vi "HFRR ADV v016 new software.vi"() -> ()   [LabVIEW 2025] (continued)
              tunnel: w2019 -> [w2034]
              i -> [w2030]
              stop <- w2029 continue-if-true
              (unwired) TRUE ("line mode (F)")
              n2041 = Read from Text File "Read File"(file (use dialog)=w2034) -> (text=w2031:string)  [unwired: 3 in, 3 out]
              n2042 = local write "Numeric 8"(w2030) -> ()
              n2043 = String Length(string=w2031) -> (length=w2033:i32)
              n2044 = Greater?(x=w2033, y=1) -> (0:w2029:bool)
            }
          }
          frame #1 {
            w2204 = FALSE ("ACTUAL   MERGE")
            # "Sample Temp"
            # "ECR"
            # "COF"
            # "Time\nCOF\nFF\nTemp"
            n2045 = case shown="True" w2077 {
              tunnel: [w2224 w2225] -> w2078
              frame False {
                n2046 = local read "string1"() -> (w2224:string)
              }
              frame True {
                n2047 = local read "String Indicator 4"() -> (w2225:string)
              }
            }
            n2048 = local read "string1 3"() -> (w2122:string)
            n2049 = String To Path(string=w2078) -> (path=w2209:path)
            n2050 = String To Path(string=w2122) -> (path=w2220:path)
            n2051 = local read "Numeric 12"() -> (w2206:i32)
            n2052 = local read "Numeric 8"() -> (w2208:i32)
            n2053 = local read "string1 2"() -> (w2123:string)
            n2054 = local read "string1 4"() -> (w2121:string)
            n2055 = Open/Create/Replace File "Open File"(file path (use dialog)=w2209) -> (refnum out=w2223:refnum<file>, error out=w2222:errorcluster)  [unwired: 5 in, 1 out]
            n2056 = Open/Create/Replace File "Open File"(file path (use dialog)=w2220) -> (refnum out=w2216:refnum<file>, error out=w2217:errorcluster)  [unwired: 5 in, 1 out]
            n2057 = for {
              N: w2208 -> [_]
              tunnel: w2223 -> [w2371]
              tunnel: w2222 -> [w2370]
              tunnel: [w2360] -> w2135 mode=indexing
              tunnel: [w2358] -> w2192 mode=indexing
              tunnel: [w2359] -> w2187 mode=indexing
              tunnel: w2204 -> [_]
              tunnel: [w2352] -> w2189 mode=indexing
              tunnel: [w2348] -> w2158 mode=indexing
              tunnel: [w2344] -> w2133 mode=indexing
              tunnel: [w2340] -> w2114 mode=indexing
              tunnel: [w2335] -> w2074 mode=indexing
              (unwired) TRUE ("line mode (F)")
              # "freq"
              # "Stroke"
              # "Time"
              # "CoF"
              # "Humidity"
              # "Temp"
              # "Air Temp"
              # "ECR"
              n2058 = Read from Text File "Read File"(file (use dialog)=w2371, error in=w2370) -> (text=w2336:string)  [unwired: 2 in, 3 out]
              n2059 = local write "String 6"(w2336) -> ()
              n2060 = String Subset(string=w2336, offset (0)=0, length (rest)=14 ("length (rest)")) -> (substring=w2364:string)
              n2061 = String Subset(string=w2336, offset (0)=35, length (rest)=9 ("length (rest)")) -> (substring=w2361:string)
              n2062 = String Subset(string=w2336, offset (0)=15, length (rest)=9 ("length (rest)")) -> (substring=w2367:string)
              n2063 = Fract/Exp String To Number(string=w2364) -> (number=w2360:dbl)  [unwired: 3 in, 1 out]
              n2064 = Fract/Exp String To Number(string=w2361) -> (number=w2359:dbl)  [unwired: 3 in, 1 out]
              n2065 = Fract/Exp String To Number(string=w2367) -> (number=w2358:dbl)  [unwired: 3 in, 1 out]
              n2066 = String Subset(string=w2336, offset (0)=85, length (rest)=9 ("length (rest)")) -> (substring=w2337:string)
              n2067 = String Subset(string=w2336, offset (0)=25, length (rest)=9 ("length (rest)")) -> (substring=w2343:string)
              n2068 = String Subset(string=w2336, offset (0)=55, length (rest)=9 ("length (rest)")) -> (substring=w2345:string)
              n2069 = String Subset(string=w2336, offset (0)=45, length (rest)=9 ("length (rest)")) -> (substring=w2351:string)
              n2070 = String Subset(string=w2336, offset (0)=65, length (rest)=9 ("length (rest)")) -> (substring=w2357:string)
              n2071 = Fract/Exp String To Number(string=w2343) -> (number=w2340:dbl)  [unwired: 3 in, 1 out]
              n2072 = Fract/Exp String To Number(string=w2337) -> (number=w2335:dbl)  [unwired: 3 in, 1 out]
              n2073 = Fract/Exp String To Number(string=w2345) -> (number=w2344:dbl)  [unwired: 3 in, 1 out]
              n2074 = Fract/Exp String To Number(string=w2351) -> (number=w2348:dbl)  [unwired: 3 in, 1 out]
              n2075 = Fract/Exp String To Number(string=w2357) -> (number=w2354:dbl)  [unwired: 3 in, 1 out]
              n2076 = Add(x=w2354, y=0.0) -> (x+y=w2352:dbl)
            }
            n2077 = for {
              N: w2206 -> [_]
              tunnel: w2217 -> [w2297]
              tunnel: w2216 -> [w2296]
              tunnel: [w2286] -> w2175 mode=indexing
              tunnel: [w2284] -> w2173 mode=indexing
              tunnel: [w2285] -> w2169 mode=indexing
              tunnel: w2204 -> [_]
              tunnel: [w2278] -> w2171 mode=indexing
              tunnel: [w2274] -> w2153 mode=indexing
              tunnel: [w2270] -> w2129 mode=indexing
              tunnel: [w2267] -> w2110 mode=indexing
              tunnel: [w2263] -> w2069 mode=indexing
              (unwired) 9 ("length (rest)")
              (unwired) 9 ("length (rest)")
              (unwired) TRUE ("line mode (F)")
              n2078 = Read from Text File "Read File"(file (use dialog)=w2296, error in=w2297) -> (text=w2264:string)  [unwired: 2 in, 3 out]
              n2079 = local write "String 8"(w2264) -> ()
              n2080 = String Subset(string=w2264, offset (0)=85) -> (substring=w2266:string)  [unwired: 1 in]
              n2081 = String Subset(string=w2264, offset (0)=35, length (rest)=9 ("length (rest)")) -> (substring=w2287:string)
              n2082 = String Subset(string=w2264, offset (0)=55, length (rest)=9 ("length (rest)")) -> (substring=w2272:string)
              n2083 = String Subset(string=w2264, offset (0)=25) -> (substring=w2268:string)  [unwired: 1 in]
              n2084 = String Subset(string=w2264, offset (0)=15, length (rest)=9 ("length (rest)")) -> (substring=w2293:string)
              n2085 = String Subset(string=w2264, offset (0)=0, length (rest)=14 ("length (rest)")) -> (substring=w2290:string)
              n2086 = String Subset(string=w2264, offset (0)=45, length (rest)=9 ("length (rest)")) -> (substring=w2277:string)
              n2087 = String Subset(string=w2264, offset (0)=65, length (rest)=9 ("length (rest)")) -> (substring=w2283:string)
              n2088 = Fract/Exp String To Number(string=w2266) -> (number=w2263:dbl)  [unwired: 3 in, 1 out]
              n2089 = Fract/Exp String To Number(string=w2287) -> (number=w2285:dbl)  [unwired: 3 in, 1 out]
              n2090 = Fract/Exp String To Number(string=w2272) -> (number=w2270:dbl)  [unwired: 3 in, 1 out]
              n2091 = Fract/Exp String To Number(string=w2268) -> (number=w2267:dbl)  [unwired: 3 in, 1 out]
              n2092 = Fract/Exp String To Number(string=w2293) -> (number=w2284:dbl)  [unwired: 3 in, 1 out]
              n2093 = Fract/Exp String To Number(string=w2290) -> (number=w2286:dbl)  [unwired: 3 in, 1 out]
              n2094 = Fract/Exp String To Number(string=w2277) -> (number=w2274:dbl)  [unwired: 3 in, 1 out]
              n2095 = Fract/Exp String To Number(string=w2283) -> (number=w2280:dbl)  [unwired: 3 in, 1 out]
              n2096 = Add(x=w2280, y=0.0) -> (x+y=w2278:dbl)
            }
            n2097 = String To Path(string=w2123) -> (path=w2221:path)
            n2098 = String To Path(string=w2121) -> (path=w2215:path)
            n2099 = local read "Numeric 11"() -> (w2205:i32)
            n2100 = local read "Numeric 13"() -> (w2207:i32)
            n2101 = Open/Create/Replace File "Open File"(file path (use dialog)=w2221) -> (refnum out=w2219:refnum<file>, error out=w2218:errorcluster)  [unwired: 5 in, 1 out]
            n2102 = Open/Create/Replace File "Open File"(file path (use dialog)=w2215) -> (refnum out=w2214:refnum<file>, error out=w2213:errorcluster)  [unwired: 5 in, 1 out]
            n2103 = for {
              N: w2205 -> [_]
              tunnel: w2219 -> [w2334]
              tunnel: w2218 -> [w2333]
              tunnel: [w2323] -> w2185 mode=indexing
              tunnel: [w2321] -> w2183 mode=indexing
              tunnel: [w2322] -> w2178 mode=indexing
              tunnel: w2204 -> [_]
              tunnel: [w2315] -> w2180 mode=indexing
              tunnel: [w2311] -> w2156 mode=indexing
              tunnel: [w2307] -> w2131 mode=indexing
              tunnel: [w2303] -> w2112 mode=indexing
              tunnel: [w2298] -> w2070 mode=indexing
              (unwired) TRUE ("line mode (F)")
              n2104 = Read from Text File "Read File"(file (use dialog)=w2334, error in=w2333) -> (text=w2299:string)  [unwired: 2 in, 3 out]
              n2105 = local write "String 7"(w2299) -> ()
              n2106 = String Subset(string=w2299, offset (0)=85, length (rest)=9 ("length (rest)")) -> (substring=w2302:string)
              n2107 = String Subset(string=w2299, offset (0)=35, length (rest)=9 ("length (rest)")) -> (substring=w2324:string)
              n2108 = String Subset(string=w2299, offset (0)=55, length (rest)=9 ("length (rest)")) -> (substring=w2310:string)
              n2109 = String Subset(string=w2299, offset (0)=25, length (rest)=9 ("length (rest)")) -> (substring=w2304:string)
              n2110 = String Subset(string=w2299, offset (0)=45, length (rest)=9 ("length (rest)")) -> (substring=w2312:string)
              n2111 = String Subset(string=w2299, offset (0)=0, length (rest)=14 ("length (rest)")) -> (substring=w2327:string)
              n2112 = String Subset(string=w2299, offset (0)=15, length (rest)=9 ("length (rest)")) -> (substring=w2330:string)
              n2113 = String Subset(string=w2299, offset (0)=65, length (rest)=9 ("length (rest)")) -> (substring=w2316:string)
              n2114 = Fract/Exp String To Number(string=w2302) -> (number=w2298:dbl)  [unwired: 3 in, 1 out]
              n2115 = Fract/Exp String To Number(string=w2324) -> (number=w2322:dbl)  [unwired: 3 in, 1 out]
              n2116 = Fract/Exp String To Number(string=w2310) -> (number=w2307:dbl)  [unwired: 3 in, 1 out]
              n2117 = Fract/Exp String To Number(string=w2304) -> (number=w2303:dbl)  [unwired: 3 in, 1 out]
              n2118 = Fract/Exp String To Number(string=w2312) -> (number=w2311:dbl)  [unwired: 3 in, 1 out]
              n2119 = Fract/Exp String To Number(string=w2327) -> (number=w2323:dbl)  [unwired: 3 in, 1 out]
              n2120 = Fract/Exp String To Number(string=w2330) -> (number=w2321:dbl)  [unwired: 3 in, 1 out]
              n2121 = Fract/Exp String To Number(string=w2316) -> (number=w2319:dbl)  [unwired: 3 in, 1 out]
              n2122 = Add(x=w2319, y=0.0) -> (x+y=w2315:dbl)
            }
            n2123 = for {
              N: w2207 -> [_]
              tunnel: w2214 -> [w2262]
              tunnel: w2213 -> [w2261]
              tunnel: [w2251] -> w2167 mode=indexing
              tunnel: [w2250] -> w2160 mode=indexing
              tunnel: w2204 -> [_]
              tunnel: [w2239] -> w2165 mode=indexing
              tunnel: [w2244] -> w2162 mode=indexing
              tunnel: [w2240] -> w2152 mode=indexing
              tunnel: [w2235] -> w2127 mode=indexing
              tunnel: [w2231] -> w2108 mode=indexing
              tunnel: [w2226] -> w2068 mode=indexing
              (unwired) 1.0 ("x")
              (unwired) TRUE ("line mode (F)")
              n2124 = Read from Text File "Read File"(file (use dialog)=w2262, error in=w2261) -> (text=w2227:string)  [unwired: 2 in, 3 out]
              n2125 = local write "String 12"(w2227) -> ()
              n2126 = String Subset(string=w2227, offset (0)=85, length (rest)=9 ("length (rest)")) -> (substring=w2229:string)
              n2127 = String Subset(string=w2227, offset (0)=35, length (rest)=9 ("length (rest)")) -> (substring=w2252:string)
              n2128 = String Subset(string=w2227, offset (0)=55, length (rest)=9 ("length (rest)")) -> (substring=w2237:string)
              n2129 = String Subset(string=w2227, offset (0)=25, length (rest)=9 ("length (rest)")) -> (substring=w2233:string)
              n2130 = String Subset(string=w2227, offset (0)=45, length (rest)=9 ("length (rest)")) -> (substring=w2242:string)
              n2131 = String Subset(string=w2227, offset (0)=15, length (rest)=9 ("length (rest)")) -> (substring=w2258:string)
              n2132 = String Subset(string=w2227, offset (0)=0, length (rest)=14 ("length (rest)")) -> (substring=w2255:string)
              n2133 = String Subset(string=w2227, offset (0)=65, length (rest)=9 ("length (rest)")) -> (substring=w2245:string)
              n2134 = Fract/Exp String To Number(string=w2229) -> (number=w2226:dbl)  [unwired: 3 in, 1 out]
              n2135 = Fract/Exp String To Number(string=w2252) -> (number=w2250:dbl)  [unwired: 3 in, 1 out]
              n2136 = Fract/Exp String To Number(string=w2237) -> (number=w2235:dbl)  [unwired: 3 in, 1 out]
              n2137 = Fract/Exp String To Number(string=w2233) -> (number=w2231:dbl)  [unwired: 3 in, 1 out]
              n2138 = Fract/Exp String To Number(string=w2242) -> (number=w2240:dbl)  [unwired: 3 in, 1 out]
              n2139 = Fract/Exp String To Number(string=w2258) -> (number=w2239:dbl)  [unwired: 3 in, 1 out]
              n2140 = Fract/Exp String To Number(string=w2255) -> (number=w2251:dbl)  [unwired: 3 in, 1 out]
              n2141 = Fract/Exp String To Number(string=w2245) -> (number=w2248:dbl)  [unwired: 3 in, 1 out]
              n2142 = Add(x=w2248, y=0.0) -> (x+y=w2244:dbl)
            }
            n2143 = Delete From Array(array=w2110, index=0) -> (array with subset deleted=w2083:dbl[])  [unwired: 1 in, 1 out]
            n2144 = Delete From Array(array=w2173, index=0) -> (array with subset deleted=w2146:dbl[])  [unwired: 1 in, 1 out]
            n2145 = Delete From Array(array=w2153, index=0) -> (array with subset deleted=w2141:dbl[])  [unwired: 1 in, 1 out]
            n2146 = Delete From Array(array=w2171, index=0) -> (array with subset deleted=w2172:dbl[])  [unwired: 1 in, 1 out]
            n2147 = call-poly <vilib>:"Mean.vi"("X"=w2083) -> ("mean"=→"КОФ2 4":dbl)  [unwired: 1 out]
            n2148 = call-poly <vilib>:"Mean.vi"("X"=w2146) -> ("mean"=→"КОФ3":dbl)  [unwired: 1 out]
            n2149 = call-poly <vilib>:"Mean.vi"("X"=w2141) -> ("mean"=→"CP3":dbl)  [unwired: 1 out]
            n2150 = Delete From Array(array=w2135, index=0) -> (array with subset deleted=w2062:dbl[])  [unwired: 1 in, 1 out]
            n2151 = Delete From Array(array=w2074, index=0) -> (array with subset deleted=w2061:dbl[])  [unwired: 1 in, 1 out]
            n2152 = Delete From Array(array=w2114, index=0) -> (array with subset deleted=w2085:dbl[])  [unwired: 1 in, 1 out]
            n2153 = Delete From Array(array=w2192, index=0) -> (array with subset deleted=w2147:dbl[])  [unwired: 1 in, 1 out]
            n2154 = Delete From Array(array=w2158, index=0) -> (array with subset deleted=w2143:dbl[])  [unwired: 1 in, 1 out]
            "array w/ subset deleted" <- w2143
            n2155 = Delete From Array(array=w2189, index=0) -> (array with subset deleted=w2190:dbl[])  [unwired: 1 in, 1 out]
            n2156 = call-poly <vilib>:"Mean.vi"("X"=w2085) -> ("mean"=→"КОФ2 2":dbl)  [unwired: 1 out]
            n2157 = call-poly <vilib>:"Mean.vi"("X"=w2147) -> ("mean"=→"КОФ1":dbl)  [unwired: 1 out]
            n2158 = Bundle "Bundle"(w2062, w2061) -> (w2067:cluster{dbl[], dbl[]})  [unwired: 1 in]
            n2159 = Bundle "Bundle"(w2062, w2190) -> (w2054:cluster{dbl[], dbl[]})  [unwired: 1 in]
            n2160 = Delete From Array(array=w2069, index=0) -> (array with subset deleted=w2057:dbl[])  [unwired: 1 in, 1 out]
            n2161 = Delete From Array(array=w2070, index=0) -> (array with subset deleted=w2059:dbl[])  [unwired: 1 in, 1 out]
            n2162 = Delete From Array(array=w2180, index=0) -> (array with subset deleted=w2181:dbl[])  [unwired: 1 in, 1 out]
            n2163 = Delete From Array(array=w2068, index=0) -> (array with subset deleted=w2055:dbl[])  [unwired: 1 in, 1 out]
            n2164 = Delete From Array(array=w2162, index=0) -> (array with subset deleted=w2163:dbl[])  [unwired: 1 in, 1 out]
            n2165 = Delete From Array(array=w2187, index=0) -> (array with subset deleted=w2093:dbl[])  [unwired: 1 in, 1 out]
            n2166 = Delete From Array(array=w2133, index=0) -> (array with subset deleted=w2089:dbl[])  [unwired: 1 in, 1 out]
            n2167 = Delete From Array(array=w2169, index=0) -> (array with subset deleted=w2091:dbl[])  [unwired: 1 in, 1 out]
            n2168 = Delete From Array(array=w2129, index=0) -> (array with subset deleted=w2087:dbl[])  [unwired: 1 in, 1 out]
            n2169 = Delete From Array(array=w2178, index=0) -> (array with subset deleted=w2092:dbl[])  [unwired: 1 in, 1 out]
            n2170 = Delete From Array(array=w2131, index=0) -> (array with subset deleted=w2088:dbl[])  [unwired: 1 in, 1 out]
            n2171 = Delete From Array(array=w2112, index=0) -> (array with subset deleted=w2084:dbl[])  [unwired: 1 in, 1 out]
            n2172 = Delete From Array(array=w2156, index=0) -> (array with subset deleted=w2142:dbl[])  [unwired: 1 in, 1 out]
            n2173 = Delete From Array(array=w2183, index=0) -> (array with subset deleted=w2144:dbl[])  [unwired: 1 in, 1 out]
            n2174 = Delete From Array(array=w2160, index=0) -> (array with subset deleted=w2090:dbl[])  [unwired: 1 in, 1 out]
            n2175 = Delete From Array(array=w2127, index=0) -> (array with subset deleted=w2086:dbl[])  [unwired: 1 in, 1 out]
            n2176 = Delete From Array(array=w2108, index=0) -> (array with subset deleted=w2082:dbl[])  [unwired: 1 in, 1 out]
            n2177 = Delete From Array(array=w2152, index=0) -> (array with subset deleted=w2140:dbl[])  [unwired: 1 in, 1 out]
            n2178 = Delete From Array(array=w2165, index=0) -> (array with subset deleted=w2145:dbl[])  [unwired: 1 in, 1 out]
            n2179 = Delete From Array(array=w2175, index=0) -> (array with subset deleted=w2058:dbl[])  [unwired: 1 in, 1 out]
            n2180 = Delete From Array(array=w2185, index=0) -> (array with subset deleted=w2060:dbl[])  [unwired: 1 in, 1 out]
            n2181 = Delete From Array(array=w2167, index=0) -> (array with subset deleted=w2056:dbl[])  [unwired: 1 in, 1 out]
            n2182 = Bundle "Bundle"(w2062, w2093) -> (w2080:cluster{dbl[], dbl[]})  [unwired: 1 in]
            n2183 = Bundle "Bundle"(w2062, w2147) -> (w2081:cluster{dbl[], dbl[]})  [unwired: 1 in]
            n2184 = Bundle "Bundle"(w2093, w2089) -> (w2095:cluster{dbl[], dbl[]})  [unwired: 1 in]
            n2185 = Bundle "Bundle"(w2058, w2057) -> (w2065:cluster{dbl[], dbl[]})  [unwired: 1 in]
            n2186 = Bundle "Bundle"(w2091, w2087) -> (w2097:cluster{dbl[], dbl[]})  [unwired: 1 in]
            n2187 = Bundle "Bundle"(w2058, w2091) -> (w2201:cluster{dbl[], dbl[]})  [unwired: 1 in]
            n2188 = Bundle "Bundle"(w2058, w2087) -> (w2125:cluster{dbl[], dbl[]})  [unwired: 1 in]
            n2189 = Bundle "Bundle"(w2058, w2146) -> (w2211:cluster{dbl[], dbl[]})  [unwired: 1 in]
            n2190 = Bundle "Bundle"(w2058, w2141) -> (w2149:cluster{dbl[], dbl[]})  [unwired: 1 in]
            n2191 = Bundle "Bundle"(w2058, w2172) -> (w2196:cluster{dbl[], dbl[]})  [unwired: 1 in]
            n2192 = Bundle "Bundle"(w2092, w2088) -> (w2096:cluster{dbl[], dbl[]})  [unwired: 1 in]
            n2193 = Bundle "Bundle"(w2060, w2059) -> (w2066:cluster{dbl[], dbl[]})  [unwired: 1 in]
            n2194 = Bundle "Bundle"(w2060, w2092) -> (w2203:cluster{dbl[], dbl[]})  [unwired: 1 in]
            n2195 = Bundle "Bundle"(w2060, w2088) -> (w2126:cluster{dbl[], dbl[]})  [unwired: 1 in]
            n2196 = Bundle "Bundle"(w2060, w2142) -> (w2150:cluster{dbl[], dbl[]})  [unwired: 1 in]
            n2197 = Bundle "Bundle"(w2060, w2144) -> (w2212:cluster{dbl[], dbl[]})  [unwired: 1 in]
            n2198 = Bundle "Bundle"(w2060, w2181) -> (w2194:cluster{dbl[], dbl[]})  [unwired: 1 in]
            n2199 = Bundle "Bundle"(w2090, w2086) -> (w2098:cluster{dbl[], dbl[]})  [unwired: 1 in]
            n2200 = Bundle "Bundle"(w2056, w2055) -> (w2064:cluster{dbl[], dbl[]})  [unwired: 1 in]
            n2201 = Bundle "Bundle"(w2056, w2090) -> (w2202:cluster{dbl[], dbl[]})  [unwired: 1 in]
            n2202 = Bundle "Bundle"(w2056, w2086) -> (w2124:cluster{dbl[], dbl[]})  [unwired: 1 in]
            n2203 = Bundle "Bundle"(w2056, w2140) -> (w2148:cluster{dbl[], dbl[]})  [unwired: 1 in]
            n2204 = Bundle "Bundle"(w2056, w2145) -> (w2210:cluster{dbl[], dbl[]})  [unwired: 1 in]
            n2205 = Bundle "Bundle"(w2056, w2163) -> (w2195:cluster{dbl[], dbl[]})  [unwired: 1 in]
            n2206 = call-poly <vilib>:"Mean.vi"("X"=w2143) -> ("mean"=→"CP1":dbl)  [unwired: 1 out]
            n2207 = call-poly <vilib>:"Mean.vi"("X"=w2084) -> ("mean"=→"КОФ2 3":dbl)  [unwired: 1 out]
            n2208 = call-poly <vilib>:"Mean.vi"("X"=w2142) -> ("mean"=→"CP2":dbl)  [unwired: 1 out]
            n2209 = call-poly <vilib>:"Mean.vi"("X"=w2144) -> ("mean"=→"КОФ2":dbl)  [unwired: 1 out]
            n2210 = call-poly <vilib>:"Mean.vi"("X"=w2082) -> ("mean"=→"КОФ2 5":dbl)  [unwired: 1 out]
            n2211 = call-poly <vilib>:"Mean.vi"("X"=w2140) -> ("mean"=→"CP4":dbl)  [unwired: 1 out]
            n2212 = call-poly <vilib>:"Mean.vi"("X"=w2145) -> ("mean"=→"КОФ4":dbl)  [unwired: 1 out]
            n2213 = Bundle "Bundle"(w2062, w2089) -> (w2053:cluster{dbl[], dbl[]})  [unwired: 1 in]
            n2214 = Bundle "Bundle"(w2062, w2143) -> (w2076:cluster{dbl[], dbl[]})  [unwired: 1 in]
            n2215 = Build Array "Build Array"(w2053, w2076) -> (w2079:cluster{dbl[], dbl[]}[])
            "XY Graph 17" <- w2079
            n2216 = Build Array "Build Array"(w2067, w2066, w2065, w2064) -> (→"Frequency ( Hz )":cluster{dbl[], dbl[]}[])
            n2217 = Build Array "Build Array"(w2095, w2096, w2097, w2098) -> (→"Air Temp ( °C ) vs Humidity ( % RH )":cluster{dbl[], dbl[]}[])
            n2218 = Build Array "Build Array"(w2080, w2203, w2201, w2202) -> (→"Air Temperature  ( °C )":cluster{dbl[], dbl[]}[])
            n2219 = Build Array "Build Array"(w2053, w2126, w2125, w2124) -> (→"Humidity ( %RH )":cluster{dbl[], dbl[]}[])
            n2220 = Build Array "Build Array"(w2081, w2212, w2211, w2210) -> (→"Coefficient Of Friction":cluster{dbl[], dbl[]}[])
            n2221 = Build Array "Build Array"(w2076, w2150, w2149, w2148) -> (→"Sample Temperature ( °C )":cluster{dbl[], dbl[]}[])
            n2222 = Build Array "Build Array"(w2054, w2194, w2196, w2195) -> (→"XY Graph 13":cluster{dbl[], dbl[]}[])
            n2223 = Bundle "Bundle"(w2062, w2085) -> (w2107:cluster{dbl[], dbl[]})  [unwired: 1 in]
            n2224 = Bundle "Bundle"(w2058, w2083) -> (w2105:cluster{dbl[], dbl[]})  [unwired: 1 in]
            n2225 = Bundle "Bundle"(w2060, w2084) -> (w2106:cluster{dbl[], dbl[]})  [unwired: 1 in]
            n2226 = Bundle "Bundle"(w2056, w2082) -> (w2104:cluster{dbl[], dbl[]})  [unwired: 1 in]
            n2227 = Build Array "Build Array"(w2107, w2106, w2105, w2104) -> (→"Stroke ( mm )":cluster{dbl[], dbl[]}[])
            n2228 = local write "XY Graph 16"(w2079) -> ()
          }
          frame #2 {
          }
          frame #3 {
            n2229 = local write "Numeric 8"(0 ("Numeric 8")) -> ()
            n2230 = local write "Numeric 11"(0 ("Numeric 11")) -> ()
            n2231 = local write "Numeric 12"(0 ("Numeric 12")) -> ()
            n2232 = local write "Numeric 13"(0 ("Numeric 13")) -> ()
            n2233 = property on="OPEN" class="Bool (strict)"("Visible"=TRUE) -> ()  [unwired: 2 in, 2 out]
            n2234 = local read "String Control 2"() -> (w2379:string)
            n2235 = local read "String Control 4"() -> (w2378:string)
            n2236 = local read "String Control 6"() -> (w2377:string)
            n2237 = local read "String Control 8"() -> (w2376:string)
            n2238 = Match Pattern(string=w2379, regular expression="Samples / cycle :- ") -> (after substring=w2393:string)  [unwired: 1 in, 3 out]
            n2239 = Match Pattern(string=w2379, regular expression="Frequency :- ") -> (after substring=w2412:string)  [unwired: 1 in, 3 out]
            n2240 = Match Pattern(string=w2378, regular expression="Samples / cycle :- ") -> (after substring=w2389:string)  [unwired: 1 in, 3 out]
            n2241 = Match Pattern(string=w2378, regular expression="Frequency :- ") -> (after substring=w2407:string)  [unwired: 1 in, 3 out]
            n2242 = Match Pattern(string=w2377, regular expression="Samples / cycle :- ") -> (after substring=w2385:string)  [unwired: 1 in, 3 out]
            n2243 = Match Pattern(string=w2377, regular expression="Frequency :- ") -> (after substring=w2402:string)  [unwired: 1 in, 3 out]
            n2244 = Match Pattern(string=w2376, regular expression="Samples / cycle :- ") -> (after substring=w2381:string)  [unwired: 1 in, 3 out]
            n2245 = Match Pattern(string=w2376, regular expression="Frequency :- ") -> (after substring=w2397:string)  [unwired: 1 in, 3 out]
            n2246 = String Subset(string=w2393, length (rest)=6 ("length (rest)")) -> (substring=w2395:string)  [unwired: 1 in]
            n2247 = String Subset(string=w2412, length (rest)=9 ("length (rest)")) -> (substring=w2414:string)  [unwired: 1 in]
            n2248 = String Subset(string=w2389, length (rest)=6 ("length (rest)")) -> (substring=w2391:string)  [unwired: 1 in]
            n2249 = String Subset(string=w2407, length (rest)=9 ("length (rest)")) -> (substring=w2409:string)  [unwired: 1 in]
            n2250 = String Subset(string=w2385, length (rest)=6 ("length (rest)")) -> (substring=w2387:string)  [unwired: 1 in]
            n2251 = String Subset(string=w2402, length (rest)=9 ("length (rest)")) -> (substring=w2404:string)  [unwired: 1 in]
            n2252 = String Subset(string=w2381, length (rest)=6 ("length (rest)")) -> (substring=w2383:string)  [unwired: 1 in]
            n2253 = String Subset(string=w2397, length (rest)=9 ("length (rest)")) -> (substring=w2399:string)  [unwired: 1 in]
            n2254 = Fract/Exp String To Number(string=w2395) -> (number=w2375:dbl)  [unwired: 3 in, 1 out]
            n2255 = Fract/Exp String To Number(string=w2414) -> (number=w2415:dbl)  [unwired: 3 in, 1 out]
            n2256 = Fract/Exp String To Number(string=w2391) -> (number=w2374:dbl)  [unwired: 3 in, 1 out]
            n2257 = Fract/Exp String To Number(string=w2409) -> (number=w2410:dbl)  [unwired: 3 in, 1 out]
            n2258 = Fract/Exp String To Number(string=w2387) -> (number=w2373:dbl)  [unwired: 3 in, 1 out]
            n2259 = Fract/Exp String To Number(string=w2404) -> (number=w2405:dbl)  [unwired: 3 in, 1 out]
            n2260 = Fract/Exp String To Number(string=w2383) -> (number=w2372:dbl)  [unwired: 3 in, 1 out]
            n2261 = Fract/Exp String To Number(string=w2399) -> (number=w2400:dbl)  [unwired: 3 in, 1 out]
            n2262 = local write "sample1"(w2375) -> ()
            n2263 = local write "freq1"(w2415) -> ()
            n2264 = local write "sample2"(w2374) -> ()
            n2265 = local write "freq2"(w2410) -> ()
            n2266 = local write "sample3"(w2373) -> ()
            n2267 = local write "freq3"(w2405) -> ()
            n2268 = local write "sample4"(w2372) -> ()
            n2269 = local write "freq 4"(w2400) -> ()
          }
        }
      }
    }
    n2270 = case shown="True" w1864 {
      selector: w1864 -> [_ w1992]
      frame False {
      }
      frame True {
        n2271 = Not(x=w1992) -> (.not. x?=w1988:bool)
        n2272 = local write "service 3"(w1988) -> ()
        n2273 = local write "OPEN 6"(w1988) -> ()
        n2274 = call <vilib>:"System Exec.vi"("wait until completion? (T)"=TRUE, "command line"="C:\\LAB-IQ\\Scar View.exe") -> ("error out"=→"error out 5":errorcluster)  [unwired: 6 in, 3 out]
      }
    }
    n2275 = case shown="\"Acquire\", Default" w1875 {
      frame "Acquire", Default {
        w2888 = 0.2 ("y")
        w2893 = 1.0 ("y")
        w2894 = 0.8 ("y")
        # "Elapsed time\ncof\nstroke\nAir temp\nTemp\nHumidity"
        n2276 = disable-structure shown="Disabled" {
          frame Disabled {
            n2277 = local read "Flag"() -> (w2911:dbl)
            n2278 = local read "RUN"() -> (w2908:bool)
            n2279 = Not(x=w2908) -> (.not. x?=w2907:bool)
            n2280 = Equal?(x=w2911, y=10.0) -> (x = y?=w2909:bool)
            n2281 = And(x=w2909, y=w2907) -> (x .and. y?=w2906:bool)
            n2282 = case shown="True" w2906 {
              frame False {
              }
              frame True {
                w2912 = FALSE ("Heater Button")
                n2283 = local write "Humidity"(w2912) -> ()
                n2284 = local write "Heater Button"(w2912) -> ()
              }
            }
          }
          frame Enabled {
          }
        }
        n2285 = disable-structure shown="Disabled" {
          frame Disabled {
            n2286 = case shown="True" {
              selector: _ -> [_ _]
              frame False {
              }
              frame True {
                w3003 = TRUE ("Heater")
                n2287 = local write "Humidity"(w3003) -> ()
                n2288 = local write "Heater Button"(w3003) -> ()
                n2289 = local read "TEST STANDARD"() -> (w3006:T3)
                n2290 = local read "TEST STANDARD"() -> (w3001:T3)
                n2291 = Equal?(x=w3006, y=enum16{"ASTM D6079", "ISO 12156", "Custom"}."ISO 12156" ("Test Standard")) -> (x = y?=w3004:bool)
                n2292 = Equal?(x=w3001, y=enum16{"ASTM D6079", "ISO 12156", "Custom"}."ASTM D6079" ("Test Standard")) -> (x = y?=w3000:bool)
                n2293 = case shown="True" w3004 {
                  frame False {
                  }
                  frame True {
                    n2294 = local write "Heater"(TRUE ("Heater")) -> ()
                    n2295 = local write "airtempflg"(FALSE ("airtempflg")) -> ()
                  }
                }
                n2296 = case shown="True" w3000 {
                  frame False {
                  }
                  frame True {
                    n2297 = local write "Heater"(FALSE ("Heater")) -> ()
                    n2298 = local write "airtempflg"(TRUE ("airtempflg")) -> ()
                  }
                }
              }
            }
          }
          frame Enabled {
          }
        }
        n2299 = stacked-sequence {
          frame #0 {
            n2300 = case shown="True" "RST FF" {
              frame False {
              }
              frame True {
                w3069 = 0.0 ("X Scale.Range:Maximum")
                n2301 = property on="Frictional Force ( N )" class="WFChart (strict)"("XScale.Maximum"=600.0 ("X Scale.Range:Maximum"), "XScale.Minimum"=w3069, "YScale.Maximum"=10.0 ("Y Scale.Range:Maximum"), "YScale.Minimum"=w3069) -> ()  [unwired: 2 in, 2 out]
              }
            }
          }
          frame #1 {
            n2302 = case shown="True" "RST TEMP" {
              frame False {
              }
              frame True {
                n2303 = property on="Temperature ( Deg C )" class="WFChart (strict)"("XScale.Minimum"=0.0 ("X Scale.Range:Minimum"), "XScale.Maximum"=600.0 ("X Scale.Range:Maximum"), "YScale.Minimum"=0.0 ("Y Scale.Range:Minimum"), "YScale.Maximum"=100.0 ("Y Scale.Range:Maximum")) -> ()  [unwired: 2 in, 2 out]
              }
            }
          }
          frame #2 {
            n2304 = case shown="True" "RSTCOF" {
              frame False {
              }
              frame True {
                n2305 = property on="Coefficient of Friction" class="WFChart (strict)"("XScale.Minimum"=0.0 ("X Scale.Range:Minimum"), "XScale.Maximum"=600.0 ("X Scale.Range:Maximum"), "YScale.Maximum"=1.0 ("X Scale.Range:Minimum"), "YScale.Minimum"=0.0 ("X Scale.Range:Minimum")) -> ()  [unwired: 2 in, 2 out]
              }
            }
          }
          frame #3 {
            n2306 = case shown="True" "RSTCOF 2" {
              frame False {
              }
              frame True {
                (unwired) 100.0 ("Y Scale.Range:Maximum")
                (unwired) 0.0 ("Y Scale.Range:Minimum")
                (unwired) 600.0 ("X Scale.Range:Maximum")
                (unwired) 0.0 ("X Scale.Range:Minimum")
              }
            }
          }
          frame #4 {
            n2307 = case shown="True" "RSTCOF 3" {
              frame False {
              }
              frame True {
                n2308 = property on="Electrical Contact Resistance ( % )" class="WFChart (strict)"("XScale.Minimum"=0.0 ("X Scale.Range:Minimum"), "XScale.Maximum"=600.0 ("X Scale.Range:Maximum"), "YScale.Minimum"=0.0 ("Y Scale.Range:Minimum"), "YScale.Maximum"=100.0 ("Y Scale.Range:Maximum")) -> ()  [unwired: 2 in, 2 out]
              }
            }
          }
        }
        n2309 = disable-structure shown="Disabled" {
          frame Disabled {
            n2310 = case shown="True" {
              selector: _ -> [_ _]
              frame False {
              }
              frame True {
                n2311 = local read "zflag 2"() -> (w2970:dbl)
                n2312 = local read "yflag"() -> (w2972:dbl)
                n2313 = Equal?(x=w2972, y=2.0 ("tflag")) -> (x = y?=w2974:bool)
                n2314 = Equal?(x=w2970, y=3.0 ("tflag")) -> (x = y?=w2973:bool)
                n2315 = And(x=w2974, y=w2973) -> (x .and. y?=w2968:bool)
                n2316 = case shown="True" w2968 {
                  frame False {
                  }
                  frame True {
                    w2999 = 0.0 ("zflag")
                    n2317 = local write "zflag"(w2999) -> ()
                    n2318 = local write "zflag 2"(w2999) -> ()
                    n2319 = Delete(path (use dialog)=path "C:/LAB-IQ-NXT/WO 2449 TT.sig" ("file path (dialog if empty)")) -> (deleted path=w2998:path)  [unwired: 4 in, 2 out]
                    n2320 = Delete(path (use dialog)=path "C:/LAB-IQ-NXT/WO 2449 TRH.sig" ("file path (dialog if empty)")) -> (deleted path=w2993:path)  [unwired: 4 in, 2 out]
                    n2321 = local read "SEN.RUN HRS"() -> (w2985:dbl)
                    n2322 = local read "SENSOR TIME"() -> (w2983:dbl)
                    n2323 = call <vilib>:"compatOverwrite.vi"("overwrite (F)"=TRUE) -> ("overwrite?"=w2975:T30)
                    n2324 = call <vilib>:"compatOverwrite.vi"("overwrite (F)"=TRUE) -> ("overwrite?"=w2979:T30)
                    n2325 = local read "Total No. of Tests"() -> (w2986:dbl)
                    n2326 = Add(x=w2983, y=w2985) -> (x+y=w2984:dbl)
                    "SEN.RUN HRS" <- w2984
                    n2327 = Open/Create/Replace File(file path (use dialog)=w2998, operation (0:open)=w2975) -> (refnum out=w2976:refnum<file>, error out=w2977:errorcluster)  [unwired: 4 in, 1 out]
                    n2328 = Open/Create/Replace File(file path (use dialog)=w2993, operation (0:open)=w2979) -> (refnum out=w2980:refnum<file>, error out=w2981:errorcluster)  [unwired: 4 in, 1 out]
                    n2329 = Deny Access(4:w2977, 6:T28."deny none" ("deny mode (2)"), 7:w2976) -> (3:w2997:refnum<file>)  [unwired: 1 out]
                    n2330 = Deny Access(4:w2981, 6:T28."deny none" ("deny mode (2)"), 7:w2980) -> (3:w2989:refnum<file>)  [unwired: 1 out]
                    n2331 = Number To Decimal String(number=w2986) -> (decimal integer string=w2994:string)  [unwired: 1 in]
                    n2332 = Number To Decimal String(number=w2984) -> (decimal integer string=w2990:string)  [unwired: 1 in]
                    n2333 = Write to Binary File(file (use dialog)=w2997, data=w2994, 5:FALSE ("prepend array or string size? (T)")) -> ()  [unwired: 3 in, 3 out]
                    n2334 = Write to Binary File(file (use dialog)=w2989, data=w2990, 5:FALSE ("prepend array or string size? (T)")) -> ()  [unwired: 3 in, 3 out]
                  }
                }
              }
            }
          }
          frame Enabled {
          }
        }
        n2335 = local read "RUN"() -> (w2897:bool)
        n2336 = local read "run replace"() -> (w2901:bool)
        n2337 = local read "run replace"() -> (w2900:bool)
        n2338 = case shown="True" w2897 {
          frame False {
            n2339 = local write "run replace"(FALSE ("run replace")) -> ()
          }
          frame True {
            "run replace" <- TRUE ("run replace")
          }
        }
        n2340 = local read "RUN"() -> (w2905:bool)
        n2341 = local read "Set Temp"() -> (w2867:dbl)
        n2342 = local read "SetTemp"() -> (w2869:dbl)
        n2343 = case shown="False" w2905 {
          tunnel: [FALSE ("TEST RUNNING") TRUE ("TEST RUNNING")] -> w2904
          frame False {
            w3088 = 0.0 ("Flag")
            n2344 = local write "Elapsed time"(0.0 ("elapsedtime")) -> ()
            n2345 = local write "Time Remaining"(w3088) -> ()
            n2346 = local write "Flag"(w3088) -> ()
            n2347 = local write "Remaining Time"(w3088) -> ()
          }
          frame True {
            n2348 = local write "Flag"(10.0 ("Flag")) -> ()
          }
        }
        n2349 = case shown="False" w2901 {
          frame False {
            n2350 = local read "zflag"() -> (→"zflag 2":dbl)
            n2351 = local write "yflag"(2.0 ("tflag")) -> ()
            n2352 = local write "FLAG 4"(0.0 ("FLAG")) -> ()
          }
          frame True {
            n2353 = local write "yflag"(1.0 ("tflag")) -> ()
            n2354 = local write "zflag"(3.0 ("zflag")) -> ()
          }
        }
        n2355 = local read "acq 2"() -> (w2899:bool)
        n2356 = local read "AIR TEMP"() -> (w2862:dbl)
        n2357 = local read "Amb temp"() -> (w2866:dbl)
        n2358 = case shown="True" "Save & Continue" {
          frame False {
          }
          frame True {
            "acq 2" <- TRUE ("acq 2")
          }
        }
        n2359 = local read "Set Rh"() -> (w2868:dbl)
        n2360 = Add(x=w2869, y=w2894) -> (x+y=w2895:dbl)
        n2361 = Subtract(x=w2869, y=w2894) -> (x-y=w2896:dbl)
        n2362 = Add(x=w2867, y=w2888) -> (x+y=w2889:dbl)
        n2363 = Subtract(x=w2867, y=w2888) -> (x-y=w2890:dbl)
        n2364 = And(x=w2899, y=w2900) -> (x .and. y?=w2898:bool)
        n2365 = Greater Or Equal?(x=w2862, y=15.0) -> (x >= y?=w2863:bool)
        "powstat" <- w2863
        n2366 = local read "Humidity ( %RH )"() -> (w2865:dbl)
        n2367 = case shown="True" "Save & Continue" {
          frame False {
          }
          frame True {
            n2368 = while {
              tunnel: "0123456789abcdefghijklmnopqrstuvwxyzABCDEFGHIJKLMNOPQRSTUVWXYZ" ("string 2") -> [w3059]
              shift-right: [w3057] -> w3052
              shift-left: "" -> [w3056]
              i -> [w3066]
              stop <- w3065 stop-if-true
              n2369 = Random Number (0-1)() -> (number: 0 to 1=w3060:dbl)
              n2370 = Multiply(x=w3060, y=62.0) -> (x*y=w3062:dbl)
              n2371 = Decrement(x="Length") -> (x-1=w3055:i16)
              n2372 = To Word Integer(number=w3062) -> (16bit integer=w3063:i16)
              n2373 = String Subset(string=w3059, offset (0)=w3063, length (rest)=1 ("length (rest)")) -> (substring=w3058:string)
              n2374 = Greater Or Equal?(x=w3066, y=w3055) -> (x >= y?=w3065:bool)
              n2375 = Concatenate Strings(w3058, w3056) -> (w3057:string)
            }
            n2376 = local write "UUID"(w3052) -> ()
          }
        }
        n2377 = In Range and Coerce(upper limit=w2895, x=w2866, lower limit=w2896) -> (In Range?=w2885:bool)  [unwired: 1 out]
        n2378 = Add(x=w2868, y=w2893) -> (x+y=w2892:dbl)
        n2379 = Subtract(x=w2868, y=w2893) -> (x-y=w2891:dbl)
        n2380 = local read "TEMP"() -> (w2864:dbl)
        n2381 = case shown="True" "Save & Continue" {
          frame False {
          }
          frame True {
            n2382 = local read "Operator ID"() -> (w3383:string)
            n2383 = local read "FILE"() -> (w3389:string)
            n2384 = String Length(string=w3389) -> (length=w3387:i32)
            n2385 = String Length(string=w3383) -> (length=w3384:i32)
            n2386 = Greater?(x=w3387, y=0) -> (0:w3386:bool)
            n2387 = Greater?(x=w3384, y=0) -> (0:w3382:bool)
            n2388 = And(x=w3386, y=w3382) -> (x .and. y?=w3381:bool)
            n2389 = case shown="True" w3381 {
              frame False {
                n2390 = stacked-sequence {
                  frame #0 {
                    n2391 = One Button Dialog(message="Please Enter a File Name and Operator ID to save data !", button name ("OK")="Ok") -> ()  [unwired: 1 out]
                  }
                  frame #1 {
                    n2392 = local write "Save & Continue"(FALSE ("OK Button")) -> ()
                  }
                }
                n2393 = local write "Save & Continue"(FALSE ("OK Button")) -> ()
              }
              frame True {
                n2394 = stacked-sequence {
                  frame #0 {
                    n2395 = local read "FILE"() -> (w3395:string)
                    n2396 = call "file check.vi"("file name in"=w3395) -> ("file name out"=w3394:string)  [unwired: 9 in, 1 out]
                    n2397 = call <vilib>:"Application Directory.vi"() -> ("Application Directory"=w3405:path)
                    n2398 = Build Path(base path=w3405, name or relative path="data") -> (appended path=w3404:path)
                    n2399 = call <vilib>:"Trim Whitespace.vi"("string"=w3394) -> ("trimmed string"=w3402:string)  [unwired: 1 in]
                    n2400 = call <vilib>:"Trim Whitespace.vi"("string"=w3394) -> ("trimmed string"=w3403:string)  [unwired: 1 in]
                    n2401 = List Folder(path=w3404) -> (folder names=w3400:string[])  [unwired: 3 in, 3 out]
                    n2402 = Match Pattern(string=w3402, regular expression="_(") -> (before substring=w3399:string)  [unwired: 1 in, 3 out]
                    n2403 = for {
                      tunnel: w3400 -> [w3414] mode=indexing
                      tunnel: w3399 -> [w3412]
                      shift-right: [w3410] -> w3397
                      shift-left: bool[] [] -> [w3411]
                      n2404 = Match Pattern(string=w3414, regular expression="_(") -> (before substring=w3413:string)  [unwired: 1 in, 3 out]
                      n2405 = Equal?(x=w3413, y=w3412) -> (x = y?=w3409:bool)
                      n2406 = case shown="True" w3409 {
                        tunnel: w3409 -> [_ w3417]
                        tunnel: w3411 -> [w3416 w3419]
                        tunnel: [w3416 w3418] -> w3410
                        frame False {
                        }
                        frame True {
                          n2407 = Insert Into Array(array=w3419, new element=w3417) -> (w3418:bool[])  [unwired: 1 in]
                        }
                      }
                    }
                    n2408 = Equal?(x=w3400, y=w3399) -> (x = y?=w3408:bool[])
                    n2409 = Or Array Elements(Boolean array=w3408) -> (logical OR=w3407:bool)
                    n2410 = Array Size(array=w3397) -> (size(s)=w3396:i32)
                    n2411 = case shown="True" w3407 {
                      tunnel: w3403 -> [_ w3427]
                      tunnel: w3396 -> [_ w3420]
                      frame False {
                      }
                      frame True {
                        n2412 = Number To Decimal String(number=w3420) -> (decimal integer string=w3423:string)  [unwired: 1 in]
                        n2413 = Search/Split String(string=w3427, search string/char (-)="_(" ("regular expression")) -> (substring before match=w3425:string)  [unwired: 1 in, 2 out]
                        n2414 = Concatenate Strings(w3425, "_(" ("regular expression"), w3423, ")" ("regular expression")) -> (w3421:string)
                        n2415 = local write "FILE"(w3421) -> ()
                      }
                    }
                  }
                  frame #1 {
                    w3429 = 0.0
                    w3442 = cluster{"y":dbl, dbl, "y":dbl}[] [] ("History Data")
                    w3443 = FALSE ("Heater Button")
                    (unwired) ")!" ("string")
                    (unwired) ")" ("string")
                    w3441 = dbl[] [] ("History Data")
                    w3447 = "\r"
                    # "C:\\WinDucom\\Data\\"
                    # "C:\\LAB-IQ-NXT\\data"
                    n2416 = local write "Humidity ( %RH )"(w3429) -> ()
                    n2417 = local write "Frequency ( Hz )"(w3429) -> ()
                    n2418 = local write "Stroke 3"(w3429) -> ()
                    n2419 = local write "speedop"(0.0 ("PIDclk 2")) -> ()
                    n2420 = local write "Set Temp 2"(65.0 ("Set Temp 2")) -> ()
                    n2421 = local write "AIR TEMP"(w3429) -> ()
                    n2422 = local write "clk"(0.0 ("clk")) -> ()
                    n2423 = local write "Stroke 4"(w3429) -> ()
                    n2424 = local write "COF 2"(w3429) -> ()
                    n2425 = local write "TEMP"(w3429) -> ()
                    n2426 = local write "ecr 3"(w3429) -> ()
                    n2427 = local write "FF 3"(w3429) -> ()
                    n2428 = local write "FF 2"(w3429) -> ()
                    n2429 = property on="Humidity ( %RH )" class="WFChart (strict)"("History Data"=w3441) -> ()  [unwired: 2 in, 2 out]
                    n2430 = property on="Coefficient of Friction" class="WFChart (strict)"("History Data"=w3441) -> ()  [unwired: 2 in, 2 out]
                    n2431 = property on="Coefficient of Friction" class="WFChart (strict)"("History Data"=w3441) -> ()  [unwired: 2 in, 2 out]
                    n2432 = property on="Frictional Force ( N )" class="WFChart (strict)"("History Data"=w3441) -> ()  [unwired: 2 in, 2 out]
                    n2433 = property on="Electrical Contact Resistance ( % )" class="WFChart (strict)"("History Data"=w3441) -> ()  [unwired: 2 in, 2 out]
                    n2434 = property on="Electrical Contact Resistance ( % )" class="WFChart (strict)"("History Data"=w3441) -> ()  [unwired: 2 in, 2 out]
                    n2435 = property on="Temperature ( Deg C )" class="WFChart (strict)"("History Data"=w3441) -> ()  [unwired: 2 in, 2 out]
                    n2436 = property on="Frictional Force ( N )" class="WFChart (strict)"("History Data"=w3441) -> ()  [unwired: 2 in, 2 out]
                    n2437 = property on="Coefficient of Friction" class="WFChart (strict)"("History Data"=w3441) -> ()  [unwired: 2 in, 2 out]
                    n2438 = property on="Frictional Force ( N )" class="WFChart (strict)"("History Data"=w3441) -> ()  [unwired: 2 in, 2 out]
                    n2439 = property on="Electrical Contact Resistance ( % )" class="WFChart (strict)"("History Data"=w3441) -> ()  [unwired: 2 in, 2 out]
                    n2440 = property on="Temperature ( Deg C )" class="WFChart (strict)"("History Data"=w3441) -> ()  [unwired: 2 in, 2 out]
                    n2441 = property on="Humidity ( %RH )" class="WFChart (strict)"("History Data"=w3441) -> ()  [unwired: 2 in, 2 out]
                    n2442 = property on="Stroke ( mm )" class="WFChart (strict)"("History Data"=w3442) -> ()  [unwired: 2 in, 2 out]
                    n2443 = property on="Stroke ( mm )" class="WFChart (strict)"("History Data"=w3442) -> ()  [unwired: 2 in, 2 out]
                    n2444 = local write "Humidity"(w3443) -> ()
                    n2445 = local write "Heater Button"(w3443) -> ()
                    n2446 = local read "FILE"() -> (w3437:string)
                    n2447 = disable-structure shown="Enabled" {
                      disable-tunnel: [w3482 _] -> w3428
                      frame Enabled {
                        n2448 = local read "NORMAL LOAD"() -> (w3482:dbl)
                      }
                      frame Disabled {
                      }
                    }
                    n2449 = call "file check.vi"("file name in"=w3437) -> ("error out"=w3440:errorcluster, "file name out"=w3434:string)  [unwired: 9 in]
                    n2450 = call "FILE PATH CREATION.vi"("error in"=w3440, "FILE NAME :"=w3434) -> ("FILE OUT"=w3433:path)  [unwired: 8 in, 1 out]
                    n2451 = Concatenate Strings(w3434, ".dgf" ("Substring")) -> (w3439:string)
                    n2452 = Concatenate Strings(w3434, ".duf" ("Substring")) -> (w3435:string)
                    n2453 = Multiply(x=w3428, y=1.0) -> (x*y=w3461:dbl)
                    n2454 = Build Path(base path=w3433, name or relative path=w3439) -> (appended path=w3432:path)
                    n2455 = Build Path(base path=w3433, name or relative path=w3435) -> (appended path=w3431:path)
                    n2456 = Number To Fractional String(number=w3461, width (-)=i16 5, precision (6)=i16 2) -> (F-format string=w3469:string)  [unwired: 1 in]
                    n2457 = local read "Fuel Discription :"() -> (w3457:string)
                    n2458 = local read "Batch Ref Num :"() -> (w3445:string)
                    n2459 = Get Date/Time String(date format (0)=enum16{"short", "long", "abbreviated"}."short") -> (date string=w3480:string, time string=w3477:string)  [unwired: 2 in]
                    n2460 = local read "Remarks :"() -> (w3456:string)
                    n2461 = Concatenate Strings("Load :- " ("Substring"), w3469, " grams ," ("Substring")) -> (w3468:string)
                    n2462 = local read "String 41"() -> (w3448:string)
                    n2463 = Concatenate Strings(w3457) -> (w3458:string)
                    n2464 = Concatenate Strings(w3445) -> (w3444:string)
                    n2465 = Concatenate Strings("tested by") -> (w3452:string)
                    n2466 = Concatenate Strings("(" ("Substring"), w3480, ")" ("Substring"), w3477) -> (w3450:string)
                    "concatenated string" <- w3450
                    n2467 = Concatenate Strings(w3456, "," ("string")) -> (w3455:string)
                    n2468 = Concatenate Strings("  TIME;      COF;       STROKE;     AIR TEMP;  TEMP;  HUMIDITY;  ECR; PID-OUT; FREQUENCY" ("Substring"), "\r") -> (w3464:string)
                    n2469 = Concatenate Strings(w3448, w3447, "Fuel Discription :-" ("Substring"), w3458, w3447, w3468, w3447, "Batch Ref Num :-" ("Substring"), w3444, w3447, " Remarks :- " ("Substring"), w3455, w3447, " Date :- " ("Substring"), w3450, w3447, "Tested By :-" ("Substring"), w3452) -> (w3462:string)
                    "REMARKS" <- w3462
                    n2470 = call <vilib>:"Write Characters To File.vi"("append to file? (new file:F)"=FALSE, "character string"=w3464, "file path (dialog if empty)"=w3432) -> ()  [unwired: 2 in, 1 out]
                    n2471 = call <vilib>:"Write Characters To File.vi"("append to file? (new file:F)"=FALSE, "character string"=w3462, "file path (dialog if empty)"=w3431) -> ()  [unwired: 2 in, 1 out]
                  }
                  frame #2 {
                    n2472 = local write "Cycles elapsed"(0 ("Cycles elapsed")) -> ()
                    n2473 = local write "cyclecount"(0 ("cyclecount")) -> ()
                    n2474 = local write "Save & Continue"(FALSE ("OK")) -> ()
                    n2475 = local write "autostrtflg"(TRUE ("autostrtflg")) -> ()
                    n2476 = local write "Save"(FALSE ("Save")) -> ()
                    n2477 = Get Date/Time In Seconds() -> (seconds since 1Jan1904=w3487:timestamp)
                    n2478 = To Double Precision Float(number=w3487) -> (double precision float=w3486:dbl)
                    n2479 = local write "acq timer"(w3486) -> ()
                    n2480 = One Button Dialog(message="Please ensure sample is mounted properly and machine is ready in all aspects for testing !", button name ("OK")="Ok") -> ()  [unwired: 1 out]
                  }
                  frame #3 {
                    n2481 = stacked-sequence {
                      frame #0 {
                        n2482 = local write "Main Dashboard Buttons"(T1."Dashboard" ("Main Dashboard Buttons")) -> ()
                        n2483 = local write "Main Tab"(T2."Acquire" ("Main Tab")) -> ()
                      }
                      frame #1 {
                        n2484 = local write "EVENT LOG"("" ("EVENT LOG")) -> ()
                      }
                      frame #2 {
                        n2485 = Wait (ms)(milliseconds to wait=u32 50) -> ()  [unwired: 1 out]
                      }
                      frame #3 {
                        n2486 = disable-structure shown="Disabled" {
                          frame Disabled {
                            n2487 = local read "EVENT LOG"() -> (w3499:string)
                            n2488 = call "Event Log.vi"("Content"="Test Details", "EVENT LOG"=w3499) -> ("EVENT LOG"=w3498:string)  [unwired: 8 in, 1 out]
                            n2489 = local write "EVENT LOG"(w3498) -> ()
                          }
                          frame Enabled {
                          }
                        }
                      }
                      frame #4 {
                        n2490 = Wait (ms)(milliseconds to wait=u32 50) -> ()  [unwired: 1 out]
                      }
                      frame #5 {
                        n2491 = local read "FILE"() -> (w3501:string)
                        n2492 = Concatenate Strings("File Name :" ("Content"), w3501) -> (w3502:string)
                        n2493 = local read "EVENT LOG"() -> (w3505:string)
                        n2494 = call "Event Log.vi"("Content"=w3502, "EVENT LOG"=w3505) -> ("EVENT LOG"=w3504:string)  [unwired: 8 in, 1 out]
                        n2495 = local write "EVENT LOG"(w3504) -> ()
                      }
                      frame #6 {
                        n2496 = Wait (ms)(milliseconds to wait=u32 50) -> ()  [unwired: 1 out]
                      }
                      frame #7 {
                        n2497 = local read "Batch Ref Num :"() -> (w3507:string)
                        n2498 = Concatenate Strings("Batch Ref No :" ("Content"), w3507) -> (w3508:string)
                        n2499 = local read "EVENT LOG"() -> (w3511:string)
                        n2500 = call "Event Log.vi"("Content"=w3508, "EVENT LOG"=w3511) -> ("EVENT LOG"=w3510:string)  [unwired: 8 in, 1 out]
                        n2501 = local write "EVENT LOG"(w3510) -> ()
                      }
                      frame #8 {
                        n2502 = Wait (ms)(milliseconds to wait=u32 50) -> ()  [unwired: 1 out]
                      }
                      frame #9 {
                        n2503 = local read "tested by"() -> (w3513:string)
                        n2504 = Concatenate Strings("Tested By :" ("Content"), w3513) -> (w3514:string)
                        n2505 = local read "EVENT LOG"() -> (w3517:string)
                        n2506 = call "Event Log.vi"("Content"=w3514, "EVENT LOG"=w3517) -> ("EVENT LOG"=w3516:string)  [unwired: 8 in, 1 out]
                        n2507 = local write "EVENT LOG"(w3516) -> ()
                      }
                      frame #10 {
                        n2508 = Wait (ms)(milliseconds to wait=u32 50) -> ()  [unwired: 1 out]
                      }
                      frame #11 {
                        n2509 = local read "TEST STANDARD"() -> (w3520:T3)
                        n2510 = case shown="\"ASTM D6079\", Default" w3520 {
                          tunnel: ["ASTM D6079" "ISO 12156" "CEC F-096-A-06" "Custom"] -> w3519
                          frame "ASTM D6079", Default {
                          }
                          frame "ISO 12156" {
                          }
                          frame "CEC F-096-A-06" {
                          }
                          frame "Custom" {
                          }
                        }
                        n2511 = Concatenate Strings("Test Standard :" ("Content"), w3519) -> (w3521:string)
                        n2512 = local read "EVENT LOG"() -> (w3524:string)
                        n2513 = call "Event Log.vi"("Content"=w3521, "EVENT LOG"=w3524) -> ("EVENT LOG"=w3523:string)  [unwired: 8 in, 1 out]
                        n2514 = local write "EVENT LOG"(w3523) -> ()
                      }
                      frame #12 {
                        n2515 = Wait (ms)(milliseconds to wait=u32 50) -> ()  [unwired: 1 out]
                      }
                      frame #13 {
                        n2516 = local read "Fuel Discription :"() -> (w3530:string)
                        n2517 = Concatenate Strings("Fuel Description :" ("Content"), w3530) -> (w3531:string)
                        n2518 = local read "EVENT LOG"() -> (w3534:string)
                        n2519 = call "Event Log.vi"("Content"=w3531, "EVENT LOG"=w3534) -> ("EVENT LOG"=w3533:string)  [unwired: 8 in, 1 out]
                        n2520 = local write "EVENT LOG"(w3533) -> ()
                      }
                      frame #14 {
                        n2521 = Wait (ms)(milliseconds to wait=u32 50) -> ()  [unwired: 1 out]
                      }
                      frame #15 {
                        n2522 = local read "Remarks :"() -> (w3536:string)
                        n2523 = Concatenate Strings("Remarks :" ("Content"), w3536) -> (w3537:string)
                        n2524 = local read "EVENT LOG"() -> (w3540:string)
                        n2525 = call "Event Log.vi"("Content"=w3537, "EVENT LOG"=w3540) -> ("EVENT LOG"=w3539:string)  [unwired: 8 in, 1 out]
                        n2526 = local write "EVENT LOG"(w3539) -> ()
                      }
                      frame #16 {
                        n2527 = Wait (ms)(milliseconds to wait=u32 50) -> ()  [unwired: 1 out]
                      }
                      frame #17 {
                        n2528 = local read "Operator ID"() -> (w3542:string)
                        n2529 = Concatenate Strings("Operator ID :" ("Content"), w3542) -> (w3544:string)
                        n2530 = local read "EVENT LOG"() -> (w3546:string)
                        n2531 = call "Event Log.vi"("Content"=w3544, "EVENT LOG"=w3546) -> ("EVENT LOG"=w3545:string)  [unwired: 8 in, 1 out]
                        n2532 = local write "EVENT LOG"(w3545) -> ()
                      }
                      frame #18 {
                        n2533 = Wait (ms)(milliseconds to wait=u32 50) -> ()  [unwired: 1 out]
                      }
                      frame #19 {
                        n2534 = disable-structure shown="Disabled" {
                          frame Disabled {
                            n2535 = local read "EVENT LOG"() -> (w3550:string)
                            n2536 = call "Event Log.vi"("Content"="Test Parameter", "EVENT LOG"=w3550) -> ("EVENT LOG"=w3549:string)  [unwired: 8 in, 1 out]
                            n2537 = local write "EVENT LOG"(w3549) -> ()
                          }
                          frame Enabled {
                          }
                        }
                      }
                      frame #20 {
                        n2538 = Wait (ms)(milliseconds to wait=u32 50) -> ()  [unwired: 1 out]
                      }
                      frame #21 {
                        n2539 = local read "Set Hz"() -> (w3554:dbl)
                        n2540 = Number To Fractional String(number=w3554, precision (6)=i16 2) -> (F-format string=w3553:string)  [unwired: 2 in]
                        n2541 = Concatenate Strings("Set Frequency [Hz] :" ("Content"), w3553) -> (w3556:string)
                        n2542 = local read "EVENT LOG"() -> (w3558:string)
                        n2543 = call "Event Log.vi"("Content"=w3556, "EVENT LOG"=w3558) -> ("EVENT LOG"=w3557:string)  [unwired: 8 in, 1 out]
                        n2544 = local write "EVENT LOG"(w3557) -> ()
                      }
                      frame #22 {
                        n2545 = Wait (ms)(milliseconds to wait=u32 50) -> ()  [unwired: 1 out]
                      }
                      frame #23 {
                        n2546 = local read "NORMAL LOAD"() -> (w3561:dbl)
                        n2547 = Number To Fractional String(number=w3561, precision (6)=i16 2) -> (F-format string=w3562:string)  [unwired: 2 in]
                        n2548 = Concatenate Strings("Applied Load [grams] :" ("Content"), w3562) -> (w3564:string)
                        n2549 = local read "EVENT LOG"() -> (w3566:string)
                        n2550 = call "Event Log.vi"("Content"=w3564, "EVENT LOG"=w3566) -> ("EVENT LOG"=w3565:string)  [unwired: 8 in, 1 out]
                        n2551 = local write "EVENT LOG"(w3565) -> ()
                      }
                      frame #24 {
                        n2552 = Wait (ms)(milliseconds to wait=u32 50) -> ()  [unwired: 1 out]
                      }
                      frame #25 {
                        n2553 = local read "Set Strk"() -> (w3569:dbl)
                        n2554 = Number To Fractional String(number=w3569, precision (6)=i16 2) -> (F-format string=w3570:string)  [unwired: 2 in]
                        n2555 = Concatenate Strings("Set Stroke [mm] :" ("Content"), w3570) -> (w3572:string)
                        n2556 = local read "EVENT LOG"() -> (w3574:string)
                        n2557 = call "Event Log.vi"("Content"=w3572, "EVENT LOG"=w3574) -> ("EVENT LOG"=w3573:string)  [unwired: 8 in, 1 out]
                        n2558 = local write "EVENT LOG"(w3573) -> ()
                      }
                      frame #26 {
                        n2559 = Wait (ms)(milliseconds to wait=u32 50) -> ()  [unwired: 1 out]
                      }
                      frame #27 {
                        n2560 = local read "Set Temp"() -> (w3577:dbl)
                        n2561 = Number To Fractional String(number=w3577, precision (6)=i16 2) -> (F-format string=w3578:string)  [unwired: 2 in]
                        n2562 = Concatenate Strings("Set Temperature [deg C] :" ("Content"), w3578) -> (w3580:string)
                        n2563 = local read "EVENT LOG"() -> (w3582:string)
                        n2564 = call "Event Log.vi"("Content"=w3580, "EVENT LOG"=w3582) -> ("EVENT LOG"=w3581:string)  [unwired: 8 in, 1 out]
